vi "Write Subscribe Set.vi"(8 "error in (no error)":errorcluster, 10 "Subscribe Set":T1, 11 "Observer in":refnum<class "Observer.lvclass">) -> (0 "error out":errorcluster, 3 "Observer out":refnum<class "Observer.lvclass">)   [LabVIEW 2024, in "Observer.lvclass"]
uses:
  Observer.lvclass
  Type Def/Subcribe Set.ctl
  Subscriber/Subscriber.lvclass
  Observer.lvclass/Observer.ctl
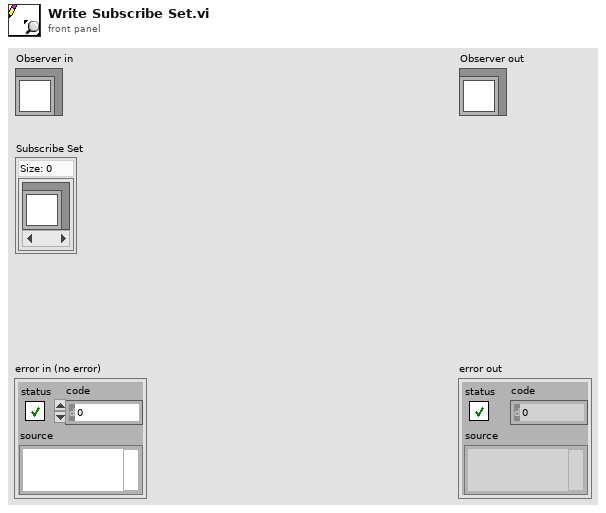
[diagram p1: front panel]
types:
  T1 = typedef "Subcribe Set.ctl" = set{refnum<class "Subscriber.lvclass">}
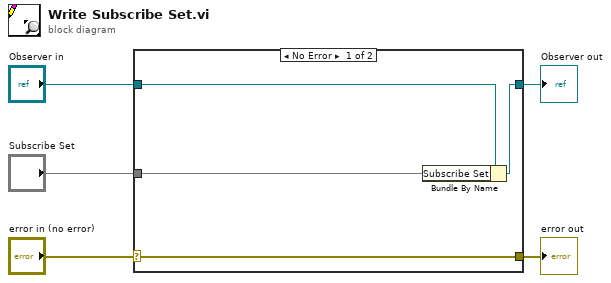
[diagram p0: block diagram]
diagram:
  n1 = case shown="No Error" "error in (no error)" {
    selector: "error in (no error)" -> [w9 w10]
    tunnel: [w9 w10] -> w4
    tunnel: [w7 w11] -> w2
    tunnel: "Observer in" -> [w8 w11]
    tunnel: "Subscribe Set" -> [w6 _]
    frame No Error {
      n2 = Bundle By Name(cluster=w8, "Subscribe Set"=w6) -> (w7:refnum<class "Observer.lvclass">)
    }
    frame Error {
    }
  }
  "error out" <- w4
  "Observer out" <- w2
